vi "myTask.vi"(8 "error in (no error)":errorcluster, 10 "stopMechanism":refnum<class "ITaskStopMechanism.lvclass">, 11 "ITask in":refnum<class "ITask.lvclass">) -> (0 "error out":errorcluster, 3 "ITask out":refnum<class "ITask.lvclass">)   [LabVIEW 2023, in "ITaskClassTemplate.lvclass"]
uses:
  ITaskClassTemplate.lvclass
  ITaskClassTemplate.lvclass/ITaskClassTemplate.ctl
  BoolNotifierStopMech/BoolNotifierStopMechanism.lvclass
  ITask/ITask.lvclass
  ITaskStopMechanism/ITaskStopMechanism.lvclass
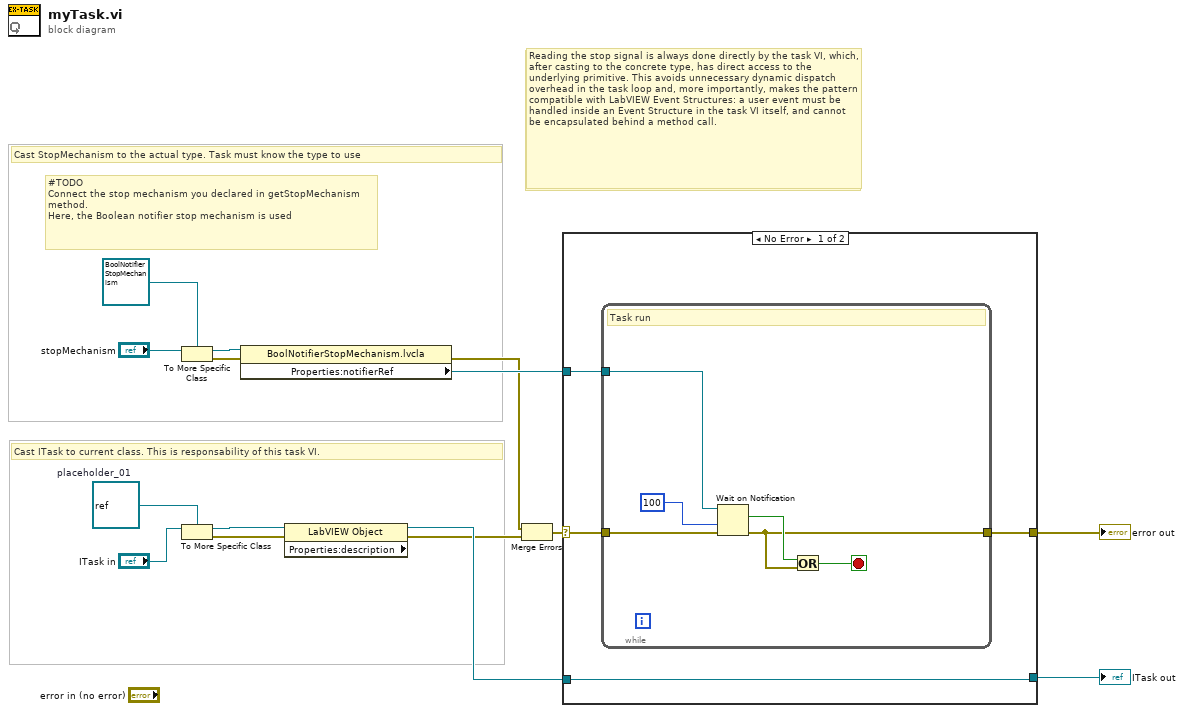
[diagram p0: block diagram]
diagram:
  w1 = refnum<class> refnum  # placeholder_01
  # "#TODO\nConnect the stop mechanism you declared in getStopMechanism method.\nHere, the Boolean notifier stop mechanism is used"
  # "The stop signal is always done directly by the task VI, which, after casting to the concrete type, has direct access to the underlying primitive. This avoids unnecessary dynamic dispatch overhead in the task loop and, more importantly, makes the pattern compatible with LabVIEW Event Structures: a user event must be handled inside an Event Structure in the task VI itself, and cannot be encapsulated behind a method call."
  # "Reading the stop signal is always done directly by the task VI, which, after casting to the concrete type, has direct access to the underlying primitive. This avoids unnecessary dynamic dispatch overhead in the task loop and, more importantly, makes the pattern compatible with LabVIEW Event Structures: a user event must be handled inside an Event Structure in the task VI itself, and cannot be encapsulated behind a method call."
  # "Cast ITask to current class. This is responsability of this task VI."
  # "Cast StopMechanism to the actual type. Task must know the type to use"
  n1 = To More Specific Class(target class=refnum<class "BoolNotifierStopMechanism.lvclass"> refnum ("TLC_Daemon.lvlib:NotifierStopMechanism.lvclass"), reference="stopMechanism") -> (specific class reference=w10:refnum<class "BoolNotifierStopMechanism.lvclass">, error out=w6:errorcluster)  [unwired: 1 in]
  n2 = To More Specific Class(target class=w1, reference="ITask in") -> (specific class reference=w11:refnum<class>, error out=w12:errorcluster)  [unwired: 1 in]
  n3 = property class="BoolNotifierStopMechanism.lvcla"(reference=w10, error in=w6) -> (error out=w4:errorcluster, "Properties:notifierRef"=w9:refnum<notifier>)  [unwired: 1 out]
  n4 = property class="LabVIEW Object" props=["Properties:description"](reference=w11, error in=w12) -> (reference out=w8:refnum<class>, error out=w5:errorcluster)  [unwired: 1 out]
  n5 = Merge Errors(w4, w5) -> (w3:errorcluster)
  n6 = case shown="No Error" w3 {
    selector: w3 -> [w17 w27]
    tunnel: w9 -> [w19 _]
    tunnel: w8 -> [w18 w26]
    tunnel: [w18 w26] -> w7
    tunnel: [w16 w27] -> w2
    frame No Error {
      n7 = while {
        tunnel: w19 -> [w25]
        tunnel: w17 -> [w21]
        tunnel: [w20] -> w16
        stop <- w22 stop-if-true
        # "Task run"
        n8 = Wait on Notification(notifier=w25, timeout in ms (-1)=100, error in (no error)=w21) -> (notification=w23:bool, error out=w20:errorcluster)  [unwired: 1 in, 2 out]
        n9 = Or(x=w23, y=w20) -> (x .or. y?=w22:bool)
      }
    }
    frame Error {
    }
  }
  "error out" <- w2
  "ITask out" <- w7
